vi "Helper.vi"(11 "Run?":bool=TRUE) -> ()   [LabVIEW 2015, in "Launcher Actor.lvclass"]
uses:
  Launcher Actor.lvclass
  Process.vi
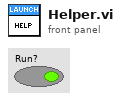
[diagram p1: front panel]
types:
  T1 = enum32{"Invalid", "Standard", "Closed", "Hidden", "Minimized", "Maximized"}
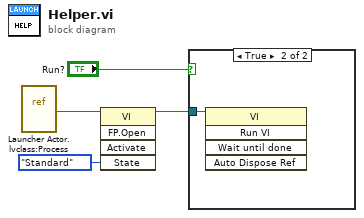
[diagram p0: block diagram]
diagram:
  n1 = vi-ref "Launcher Actor.lvclass:Process.vi"() -> (w4:refnum<vi>)
  n2 = invoke class="VI" method="FP.Open"(reference=w4, "State"=T1."Standard") -> (reference out=w2:refnum<vi>)  [unwired: 3 in, 4 out]
  n3 = case shown="True" "Run?" {
    tunnel: w2 -> [_ w5]
    frame False {
    }
    frame True {
      n4 = invoke class="VI" method="Run VI"(reference=w5) -> ()  [unwired: 4 in, 5 out]
    }
  }
